vi "relative access path.vi"(11 "Oauth2.Google":refnum<class "Oauth2.Google.lvclass">) -> (1 "Token Access Path":string, 2 "Authorization Path":string)   [LabVIEW 2020, in "Oauth2.Google.lvclass"]
uses:
  Oauth2.Google.lvclass
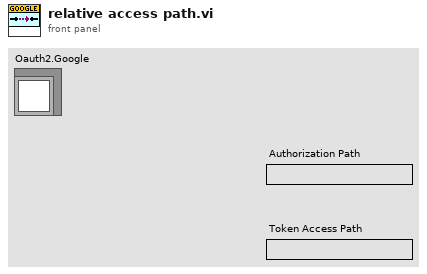
[diagram p1: front panel]
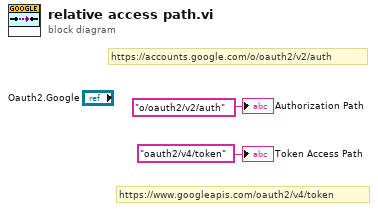
[diagram p0: block diagram]
diagram:
  # "https://www.googleapis.com/oauth2/v4/token"
  # "https://accounts.google.com/o/oauth2/v2/auth"
  "Authorization Path" <- "o/oauth2/v2/auth" ("Authorization Path")
  "Token Access Path" <- "oauth2/v4/token" ("Authorization Path")
